vi "Create REST Client.vi"(4 "Default Headers ([JSON])":T1[](array[typedef])=[{"header"="Content-Type", "value"="application/json"}], 5 "REST Client in":refnum<class "REST Client.lvclass">, 6 "Verify Server(true)":bool=TRUE, 7 "Cookie File":path, 8 "error in (no error)":errorcluster, 9 "Authentication":cluster{"Username":string, "Password":string}, 10 "Escape URLs (true)":bool=TRUE, 11 "Base URL":string) -> (0 "error out":errorcluster, 3 "REST Client out":refnum<class "REST Client.lvclass">)   [LabVIEW 2020, in "REST Client.lvlib" / "REST Client.lvclass"]
doc: "The VI provides multiple arguments for defining how to create the JKI REST Client instance.\n\n<b>Base URL</b> specifies the base URL to be used for the HTTP requests.\n\n<b>Escape URLs</b> when true instruct the REST Client to escape all URLs before executing the requests. If you have already escaped the URLs, set this to false.\n\n<b>Authentication</b> allows setting the username and password for services that use HTTP authentication.\n\n<b>Verify Server</b> when true instructs the REST Client to validate the certificate of the server when HTTPS protocol is being used.\n\n<b>Default Headers</b> specifies an array of headers to be used with every requests. Defaults to application/json content type.\n\n<b>Cookie File</b> specifies a file path to be used for cookies."
uses:
  REST Client.lvclass
  HTTP Header.ctl
  REST Client.lvclass/REST Client.ctl
  <vilib>/VIPM Community/HTTP Client Plugin - Base/Classes/Abstract HTTP Client/Abstract HTTP Client.lvclass
  <vilib>/VIPM Community/HTTP Client Plugin - Base/Classes/LabVIEW HTTP Client/LabVIEW HTTP Client.lvclass
  C:/Program Files/National Instruments/LabVIEW 2020/vi.lib/VIPM Community/HTTP Client Plugin - Base/Classes/LabVIEW HTTP Client/LabVIEW HTTP Client.lvclass
  C:/Program Files/National Instruments/LabVIEW 2020/vi.lib/VIPM Community/HTTP Client Plugin - Base/Classes/Abstract HTTP Client/Abstract HTTP Client.lvclass
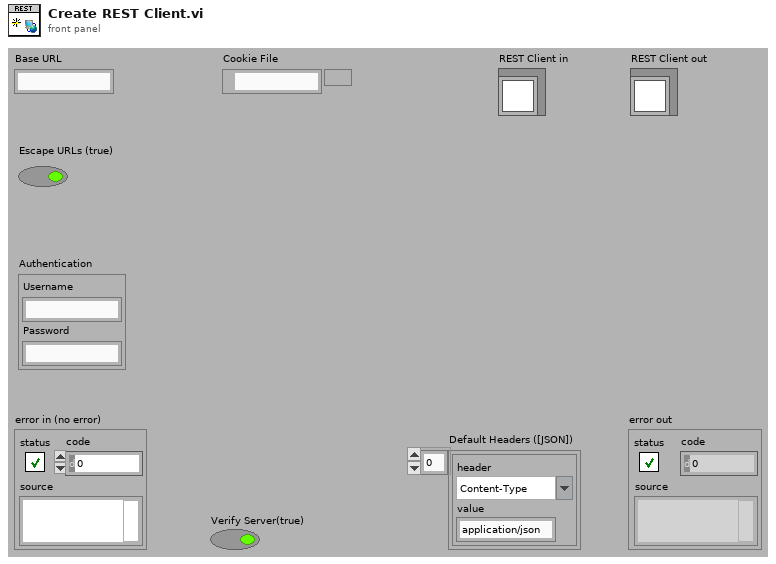
[diagram p1: front panel]
types:
  T1 = typedef "REST Client.lvlib/REST Client.lvclass/HTTP Header.ctl" = cluster{"header":string, "value":string}
  T2 = cluster{"Client Handle":refnum<class "Abstract HTTP Client.lvclass">, "Default Headers ([JSON])":T1[]}
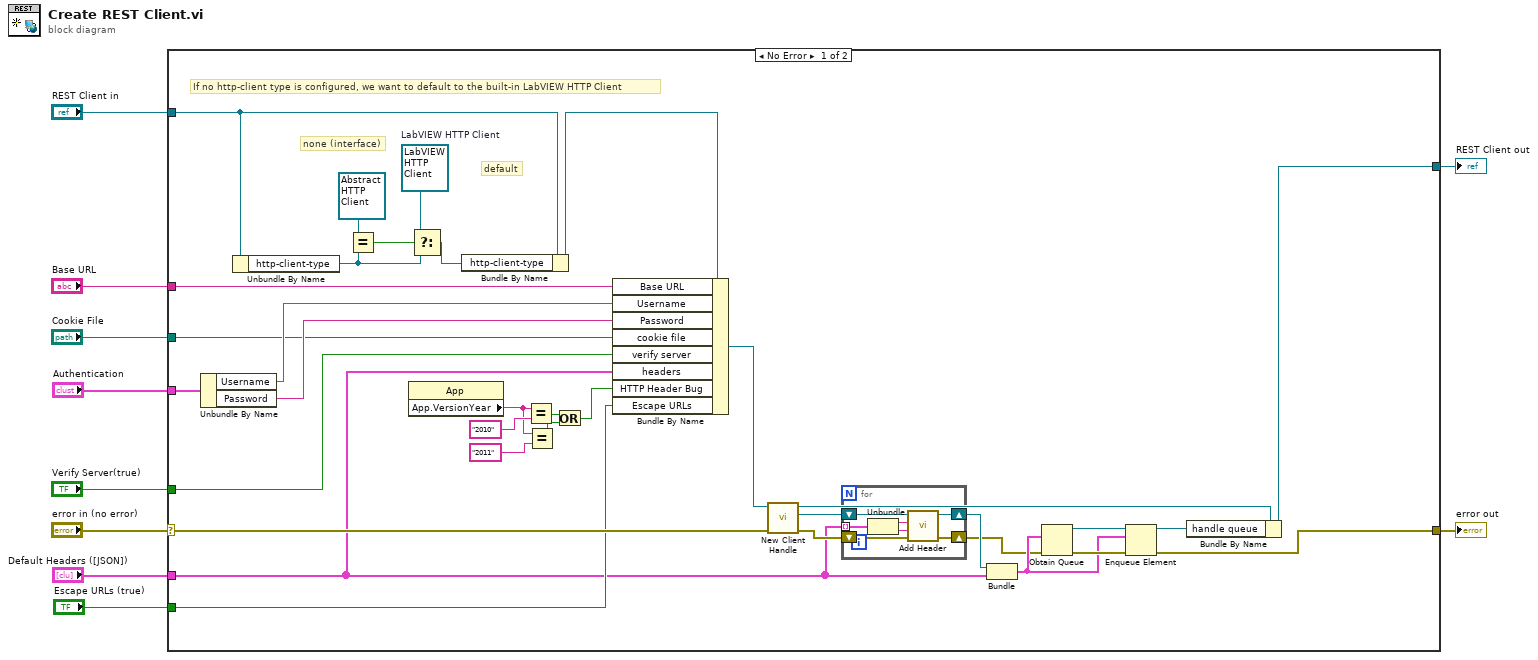
[diagram p0: block diagram]
diagram:
  n1 = case shown="No Error" "error in (no error)" {
    selector: "error in (no error)" -> [w43 w53]
    tunnel: [w39 w53] -> w9
    tunnel: [w24 w52] -> w7
    tunnel: "REST Client in" -> [w11 w52]
    tunnel: "Cookie File" -> [w27 _]
    tunnel: "Verify Server(true)" -> [w42 _]
    tunnel: "Default Headers ([JSON])" -> [w18 _]
    tunnel: "Authentication" -> [w30 _]
    tunnel: "Base URL" -> [w44 _]
    tunnel: "Escape URLs (true)" -> [w31 _]
    frame No Error {
      w15 = refnum<class "LabVIEW HTTP Client.lvclass"> refnum  # LabVIEW HTTP Client
      # "none (interface)"
      # "default"
      # "If no http-client type is configured, we want to default to the built-in LabVIEW HTTP Client"
      n2 = Unbundle By Name(w30) -> ("Username"=w29:string, "Password"=w28:string)
      n3 = Unbundle By Name(w11) -> ("http-client-type"=w14:refnum<class "Abstract HTTP Client.lvclass">)
      n4 = Equal?(x=refnum<class "Abstract HTTP Client.lvclass"> refnum ("http-client-type"), y=w14) -> (x = y?=w16:bool)
      n5 = property class="App"() -> ("App.VersionYear"=w34:string)  [unwired: 2 in, 2 out]
      n6 = Select(t=w15, s=w16, f=w14) -> (s? t:f=w13:refnum<class "Abstract HTTP Client.lvclass">)
      n7 = Bundle By Name(cluster=w11, "http-client-type"=w13) -> (w12:refnum<class "REST Client.lvclass">)
      n8 = Equal?(x=w34, y="2010") -> (x = y?=w36:bool)
      n9 = Equal?(x=w34, y="2011") -> (x = y?=w35:bool)
      n10 = Or(x=w36, y=w35) -> (x .or. y?=w32:bool)
      n11 = Bundle By Name(cluster=w12, "Base URL"=w44, "Username"=w29, "Password"=w28, "cookie file"=w27, "verify server"=w42, "headers"=w18, "HTTP Header Bug"=w32, "Escape URLs"=w31) -> (w26:refnum<class "REST Client.lvclass">)
      n12 = call "New Client Handle.vi"("error in (no error)"=w43, "REST Client in"=w26) -> ("error out"=w20:errorcluster, "Client Handle"=w22:refnum<class "Abstract HTTP Client.lvclass">, "REST Client out"=w25:refnum<class "REST Client.lvclass">)  [unwired: 7 in]
      n13 = for {
        shift-right: [w45] -> w19
        shift-left: w20 -> [w46]
        shift-right: [w47] -> w21
        shift-left: w22 -> [w50]
        tunnel: w18 -> [w51] mode=indexing
        n14 = Unbundle(w51) -> ("header"=w49:string, "value"=w48:string)
        n15 = call-dynamic "Add Header.vi"("error in (no error)"=w46, "value"=w48, "header"=w49, "HTTP Client Abstract in"=w50) -> ("error out"=w45:errorcluster, "HTTP Client Abstract out"=w47:refnum<class "Abstract HTTP Client.lvclass">)  [unwired: 6 in]
      }
      n16 = Bundle("Client Handle"=w21, "Default Headers ([JSON])"=w18) -> (w38:T2)  [unwired: 1 in]
      n17 = Obtain Queue(element data type=w38, error in (no error)=w19) -> (queue out=w41:refnum<queue>, error out=w40:errorcluster)  [unwired: 3 in, 1 out]
      n18 = Enqueue Element(queue=w41, element=w38, error in (no error)=w40) -> (queue out=w23:refnum<queue>, error out=w39:errorcluster)  [unwired: 1 in, 1 out]
      n19 = Bundle By Name(cluster=w25, "handle queue"=w23) -> (w24:refnum<class "REST Client.lvclass">)
    }
    frame Error {
    }
  }
  "error out" <- w9
  "REST Client out" <- w7
